vi "RPC General Send Request.vi"(6 "encrypt (false)":bool, 8 "error in (no error)":errorcluster, 9 "time limit (60s)":dbl=60.0, 10 "request":u8[](array[numeric]), 11 "BLE address in":string) -> (0 "error out":errorcluster, 3 "BLE address out":string)   [LabVIEW 2017]
uses:
  nimble_sensor.dll
  <vilib>/addons/Bluetooth Sensing/Bluetooth Sensing.lvlib
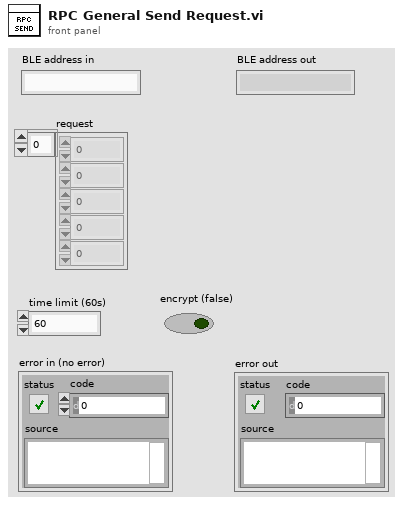
[diagram p1: front panel]
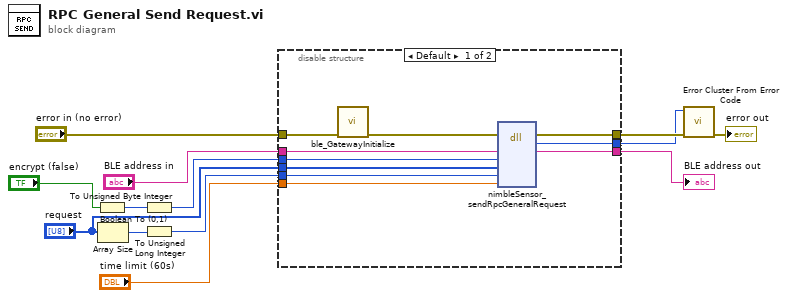
[diagram p0: block diagram]
diagram:
  n1 = Boolean To (0,1)(Boolean="encrypt (false)") -> (0, 1=w5:i16)
  n2 = Array Size(array="request") -> (size(s)=w6:i32)
  n3 = To Unsigned Byte Integer(number=w5) -> (unsigned 8bit integer=w3:u8)
  n4 = To Unsigned Long Integer(number=w6) -> (unsigned 32bit integer=w2:u32)
  n5 = disable-structure shown="Default" {
    disable-tunnel: "BLE address in" -> [w23 _]
    disable-tunnel: "time limit (60s)" -> [w22 _]
    disable-tunnel: [w21 _] -> w11
    disable-tunnel: [w20 w24] -> w9
    disable-tunnel: [w19 _] -> w8
    disable-tunnel: "request" -> [w18 _]
    disable-tunnel: "error in (no error)" -> [w15 w24]
    disable-tunnel: w3 -> [w17 _]
    disable-tunnel: w2 -> [w16 _]
    frame condition #0 (active) {
      n6 = call <vilib>:"ble_GatewayInitialize.vi"("error in (no error)"=w15) -> ("error out"=w14:errorcluster)  [unwired: 10 in]
      n7 = dll-call lib="nimble_sensor.*" fn="nimbleSensor_sendRpcGeneralRequest"(error in=w14, "address"=w23, "encrypt"=w17, "payload"=w18, "size"=w16, "timeLimit"=w22) -> (error out=w20:errorcluster, "return type"=w19:i32, "address"=w21:string)  [unwired: 6 in, 1 out]
    }
    frame condition #1 {
    }
  }
  "BLE address out" <- w11
  n8 = call <vilib>:"Error Cluster From Error Code.vi"("error in (no error)"=w9, "error code (0)"=w8) -> ("error out"=→"error out":errorcluster)  [unwired: 7 in]
